vi "Control Definition.vi"() -> ()   [LabVIEW 2013, in "SGDV_Ctrl_v13_lib.lvlib"]
uses:
  SGDV_Ctrl_v13_lib.lvlib
  Servo Drive and  Motor Paras.ctl
  PID Paras.ctl
  Pos Ctrl Paras.ctl
  Motor Coefficients.ctl
  Init Motor Data.ctl
panel:
  in  "Init Motor Data":T1
  in  "Motor Coefficients":T2={"Vel-Coefficient"=2.915, "Enc-Coefficient"=0.1, "Reduction-Ratio"=1.0}
  in  "Pos Ctrl Paras":T3={"Tolerance(deg)"=0.5, "Loop Time(ms)"=10, "Min Frequency(hz)"=40.0} {"Min Frequency(hz)" format="%#_13g"}
  in  "PID Paras":T4={"Output Range(deg/s)"={"output high"=720.0, "output low"=-720.0}, "PID gains"={"proportional gain (Kc)"=6.5, "integral time (Ti, min)"=0.0075, "derivative time (Td, min)"=0.0005}} {"PID gains"."derivative time (Td, min)" format="%.4f"; "PID gains"."integral time (Ti, min)" format="%.4f"; "PID gains"."proportional gain (Kc)" format="%.4f"; "Output Range(deg/s)"."output low" format="%.2f"; "Output Range(deg/s)"."output high" format="%.2f"}
  in  "Servo Drive and  Motor Paras":T5={"Encoder Output Pulses"=900.0, "Gear Ratio(Numerator)"=1000.0, "Gear Ratio(Denominator)"=1.0, "Reduction Ratio"=1.0} {"Gear Ratio(Denominator)" format="%#_10g"}
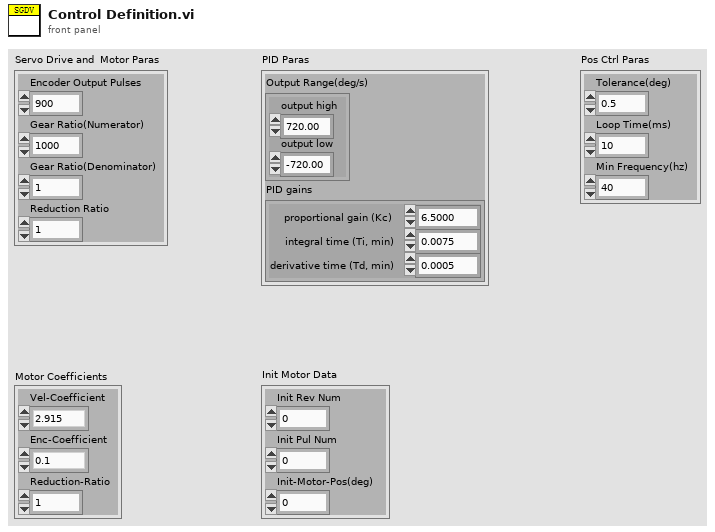
[diagram p1: front panel]
types:
  T1 = typedef "SGDV_Ctrl_v13_lib.lvlib/Init Motor Data.ctl" = cluster{"Init Rev Num":i32, "Init Pul Num":i32, "Init-Motor-Pos(deg)":dbl}
  T2 = typedef "SGDV_Ctrl_v13_lib.lvlib/Motor Coefficients.ctl" = cluster{"Vel-Coefficient":dbl, "Enc-Coefficient":dbl, "Reduction-Ratio":dbl}
  T3 = typedef "SGDV_Ctrl_v13_lib.lvlib/Pos Ctrl Paras.ctl" = cluster{"Tolerance(deg)":dbl, "Loop Time(ms)":u32, "Min Frequency(hz)":dbl}
  T4 = typedef "SGDV_Ctrl_v13_lib.lvlib/PID Paras.ctl" = cluster{"Output Range(deg/s)":cluster{"output high":dbl, "output low":dbl}, "PID gains":cluster{"proportional gain (Kc)":dbl, "integral time (Ti, min)":dbl, "derivative time (Td, min)":dbl}}
  T5 = typedef "SGDV_Ctrl_v13_lib.lvlib/Servo Drive and  Motor Paras.ctl" = cluster{"Encoder Output Pulses":dbl, "Gear Ratio(Numerator)":dbl, "Gear Ratio(Denominator)":dbl, "Reduction Ratio":dbl}
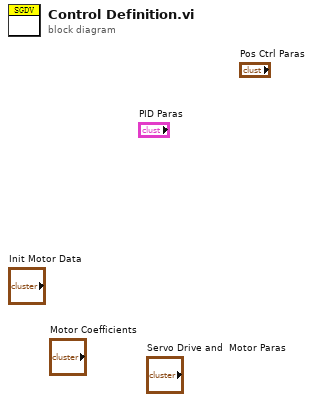
[diagram p0: block diagram]
diagram:
